vi "ManualTest_Program_with_RFmx.vi"() -> ()   [LabVIEW 2014]
uses:
  15_DataManagement/Device_Resources.ctl
panel:
  in  "Device Resources":T1={"RFSG Resource in"="VST", "RFSA Resource in"="VST", "RFmx Resource in"="VST"}
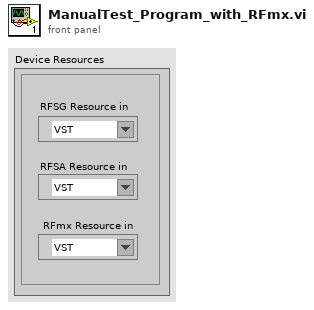
[diagram p1: front panel]
types:
  T1 = typedef "Device_Resources.ctl" = cluster{"RFSG Resource in":refnum<k15>, "RFSA Resource in":refnum<k15>, "RFmx Resource in":refnum<k15>}
  T2 = typedef "Message_Queues.ctl" = cluster{"RFSG_QTx":refnum<queue>, "RFSG_QRx":refnum<queue>, "RFSA_QTx":refnum<queue>, "RFSA_QRx":refnum<queue>, "SysLog":refnum<queue>, "RFSA_Data":refnum<queue>, "RFmx_QTx":refnum<queue>, "RFmx_QRx":refnum<queue>, "RFmx_Data":refnum<queue>}
  T3 = enum32{"Invalid", "Standard", "Closed", "Hidden", "Minimized", "Maximized"}
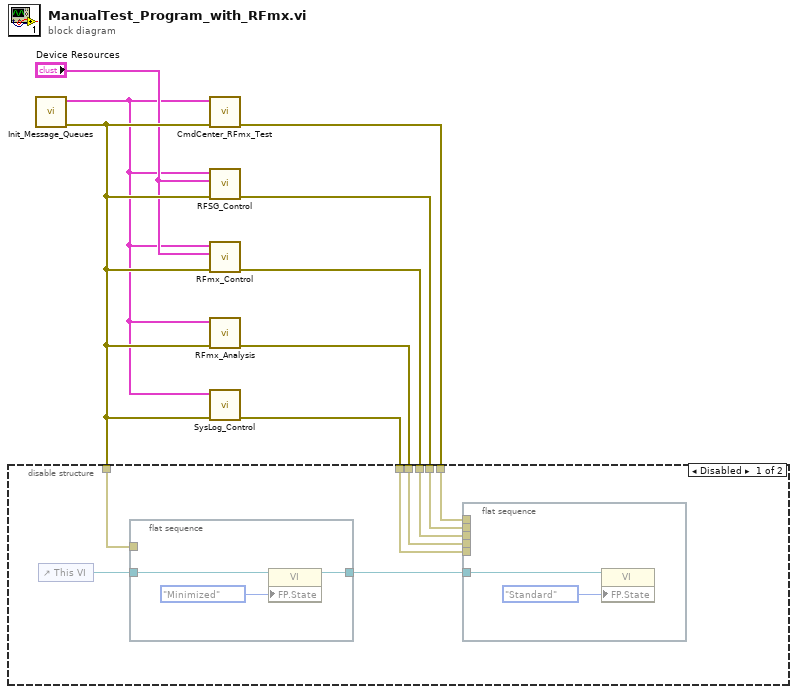
[diagram p0: block diagram]
diagram:
  n1 = call "Init_Message_Queues.vi"() -> ("error out"=w5:errorcluster, "Queue_Out"=w3:T2)  [unwired: 10 in]
  n2 = call "CmdCenter_RFmx_Test.vi"("error in (no error)"=w5, "Message_Queues"=w3) -> ("error out"=w6:errorcluster)  [unwired: 9 in]
  n3 = call "RFSG_Control.vi"("error in (no error)"=w5, "Device Resources"="Device Resources", "Message_Queues"=w3) -> ("error out"=w7:errorcluster)  [unwired: 8 in]
  n4 = call "RFmx_Control.vi"("error in (no error)"=w5, "Device Resources"="Device Resources", "Message_Queues"=w3) -> ("error out"=w2:errorcluster)  [unwired: 8 in]
  n5 = call "RFmx_Analysis.vi"("error in (no error)"=w5, "Message_Queues"=w3) -> ("error out"=w1:errorcluster)  [unwired: 9 in]
  n6 = call "SysLog_Control.vi"("error in (no error)"=w5, "Message_Queues"=w3) -> ("error out"=w8:errorcluster)  [unwired: 9 in]
  n7 = disable-structure shown="Disabled" {
    disable-tunnel: w8 -> [w14 _]
    disable-tunnel: w7 -> [w13 _]
    disable-tunnel: w6 -> [w12 _]
    disable-tunnel: w5 -> [w11 _]
    disable-tunnel: w2 -> [w10 _]
    disable-tunnel: w1 -> [w9 _]
    frame Disabled {
      n8 = control-ref of="This VI"() -> (w16:refnum<vi>)
      n9 = flat-sequence {
        tunnel: w16 -> [w22]
        tunnel: w11 -> [_]
        tunnel: [w20] -> w15
        frame #0 {
          n10 = property class="VI"(reference=w22, "FP.State"=T3."Minimized" ("Front Panel Window:State")) -> (reference out=w20:refnum<vi>)  [unwired: 1 in, 1 out]
        }
      }
      n11 = flat-sequence {
        tunnel: w15 -> [w19]
        tunnel: w10 -> [_]
        tunnel: w9 -> [_]
        tunnel: w14 -> [_]
        tunnel: w13 -> [_]
        tunnel: [w17] -> _
        tunnel: w12 -> [w17]
        frame #0 {
          n12 = property class="VI"(reference=w19, "FP.State"=T3."Standard" ("Front Panel Window:State")) -> ()  [unwired: 1 in, 2 out]
        }
      }
    }
    frame Enabled {
    }
  }
